vi "editDevPopup.vi"(10 "Device in":T1) -> (2 "Device out":T1, 3 "Abbrechen out":bool)   [LabVIEW 2013, in "DataCreation.lvlib"]
uses:
  lib/DataCreation.lvlib
panel:
  in  "Abbrechen":bool
  in  "OK":bool
  in  "Datum letzter Kalibrierung":string
  in  "Seriennummer":string
  in  "Modell":string
  in  "Hersteller":string
  # "Datenbankeintrag\nbearbeiten"
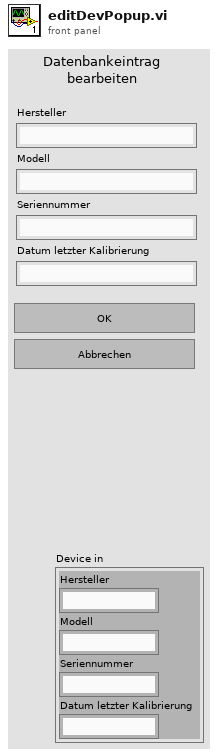
[diagram p1: front panel]
types:
  T1 = cluster{"Hersteller":string, "Modell":string, "Seriennummer":string, "Datum letzter Kalibrierung":string}
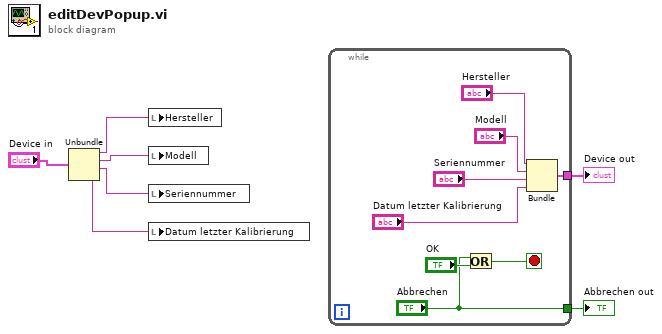
[diagram p0: block diagram]
diagram:
  n1 = Unbundle("Device in") -> ("Hersteller"=w4:string, "Modell"=w3:string, "Seriennummer"=w2:string, "Datum letzter Kalibrierung"=w1:string)
  n2 = local write "Hersteller"(w4) -> ()
  n3 = local write "Modell"(w3) -> ()
  n4 = local write "Seriennummer"(w2) -> ()
  n5 = local write "Datum letzter Kalibrierung"(w1) -> ()
  n6 = while {
    tunnel: ["Abbrechen"] -> w7
    tunnel: [w11] -> w6
    stop <- w10 stop-if-true
    n7 = Or(x="Abbrechen", y="OK") -> (x .or. y?=w10:bool)
    n8 = Bundle("Hersteller"="Hersteller", "Modell"="Modell", "Seriennummer"="Seriennummer", "Datum letzter Kalibrierung"="Datum letzter Kalibrierung") -> (w11:T1)  [unwired: 1 in]
  }
  "Abbrechen out" <- w7
  "Device out" <- w6
